vi "Elemente auswerten.vi"(7 "GObject (Eingang)":refnum<vi>, 8 "Fehler (Eingang, kein Fehler)":errorcluster, 9 "Sprachauswahl":u16, 10 "all rows":string[][](array[string]), 11 "ClassID":u32) -> (0 "error out":errorcluster, 1 "Sprachauswahl out":u16, 2 "all rows out":string[][](array[string]), 3 "ClassID out":u32, 4 "Cluster Elemente[]":refnum<vi>[](array[refnum]), 5 "Strings [4]":string[](array[string]))   [LabVIEW 2020, in "Sprachverwaltung.lvlib"]
uses:
  Sprachverwaltung.lvlib
panel:
  # "3 Generic \n4 Decoration \n5 Text \n6 Control \n7 ColorBox \n8 Boolean \n9 RefNum \n10 Variant \n11 Path \n12 ListBox \n13 Table \n14 Array \n15 Picture \n16 ActiveXContainer \n17 Numeric \n18 Digital \n19 NamedNumeric \n20 ColorRamp \n21 Slide \n22 GraphOrChart \n23 WaveformChart \n24 WaveformGraph \n25 IntensityChart \n26 IntensityGraph \n27 String \n28 IOName \n29 ComboBox \n30 Cluster \n31 Panel \n32 Knob \n33 NumWithScale \n34 Ring \n35 Enum \n36 GObject \n37 Plot \n38 Cursor \n39 NumericText \n40 Scale \n41 ColorScale \n42 GraphScale \n43 ColorGraphScale \n44 TypedRefNum \n45 OldKnobScale \n46 MCListbox \n47 MeasureData \n48 BVTag \n49 DAQName \n50 VISAName \n51 IVIName \n52 SlideScale \n54 Page \n55 TabControl \n56 ConPane"
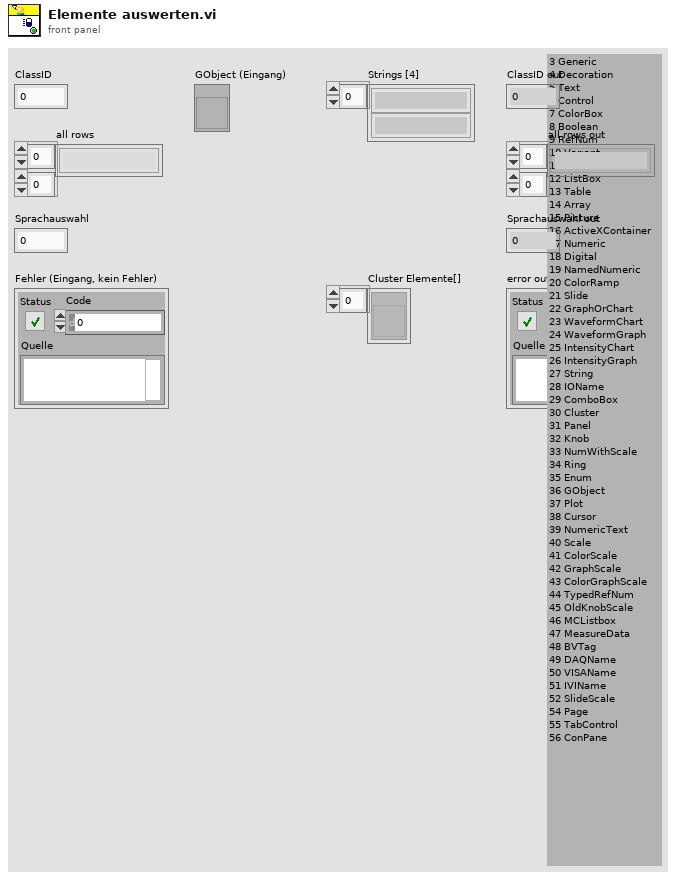
[diagram p1: front panel]
types:
  T1 = typedef "LVStringsAndValuesArrayTypeDef.ctl" = cluster{"String":string, "Value":ext}[]
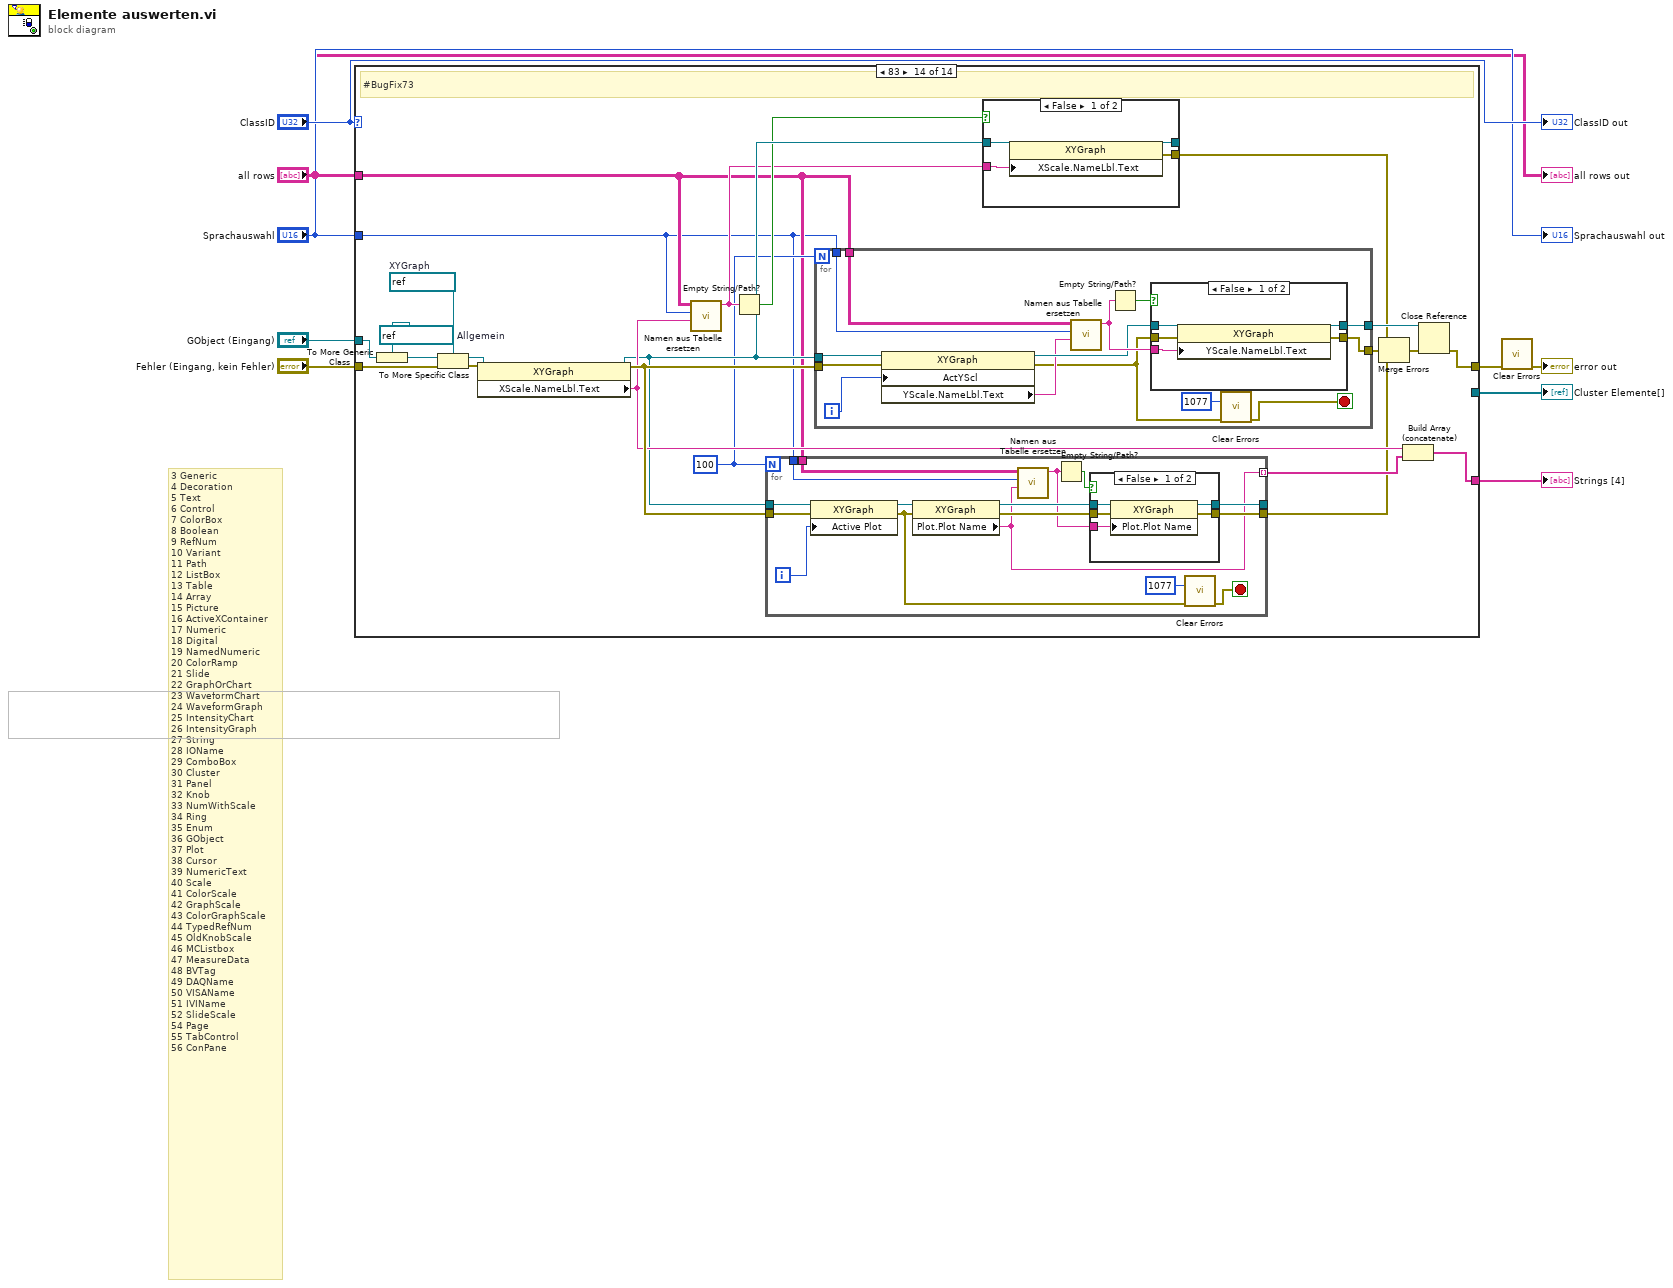
[diagram p0: block diagram]
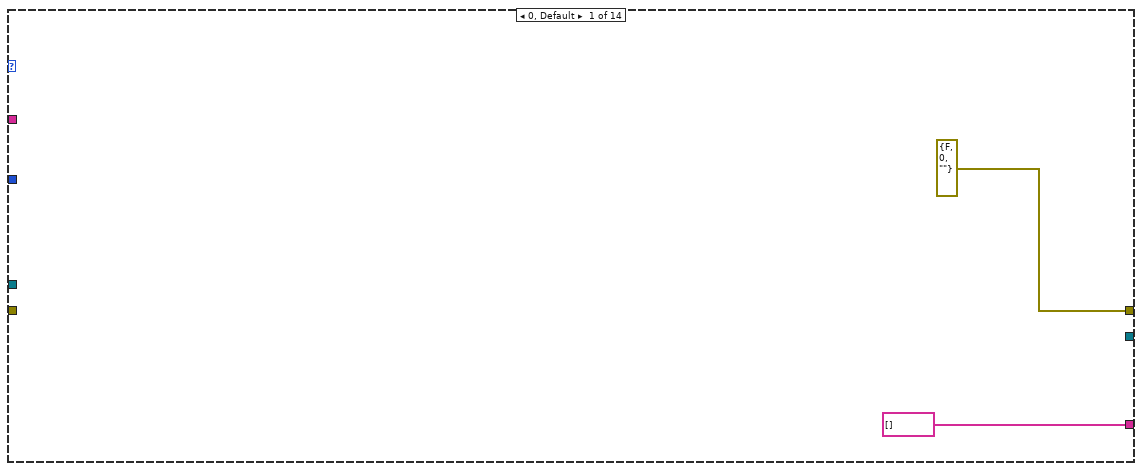
[diagram p2: hidden frame]
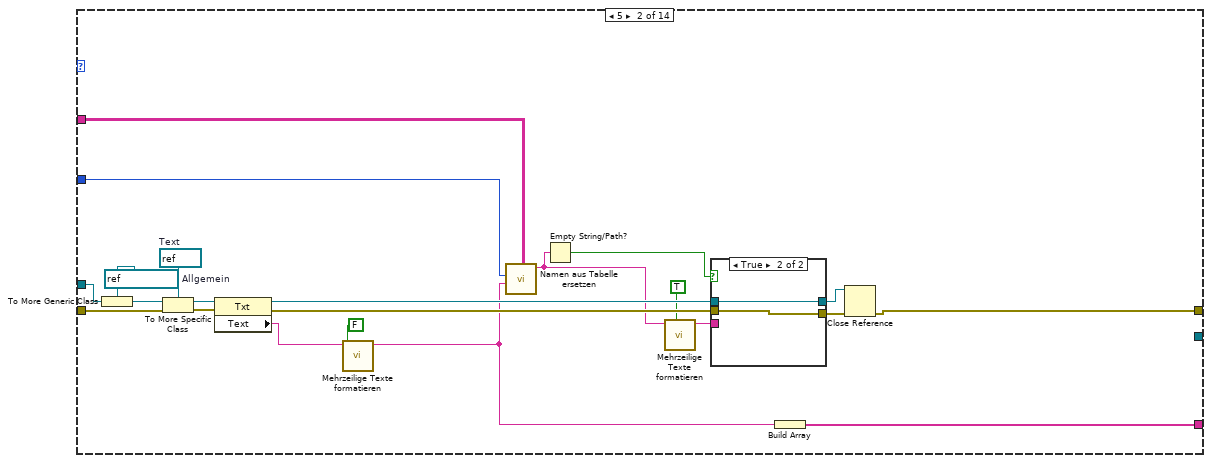
[diagram p3: hidden frame]
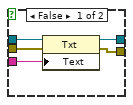
[diagram p4: hidden frame]
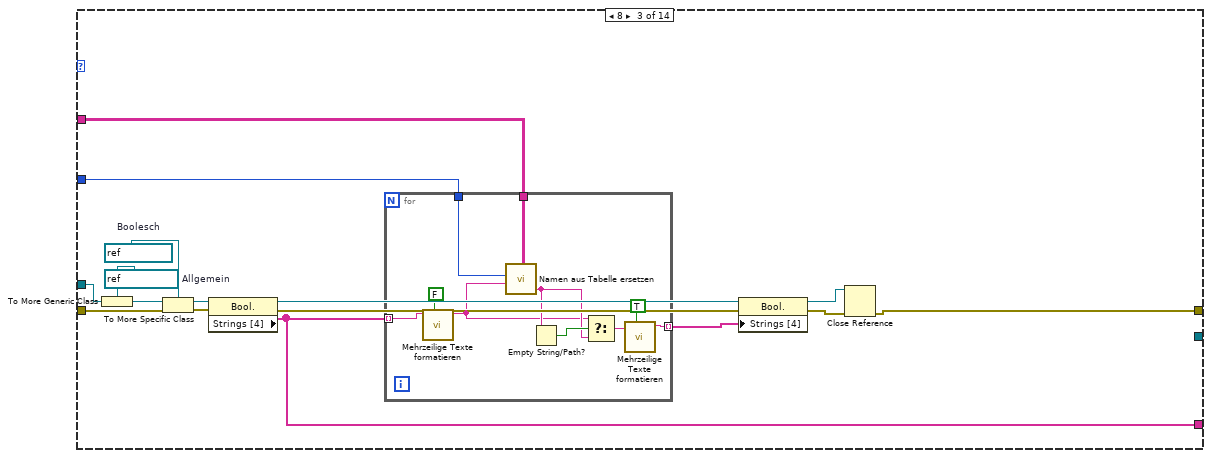
[diagram p5: hidden frame]
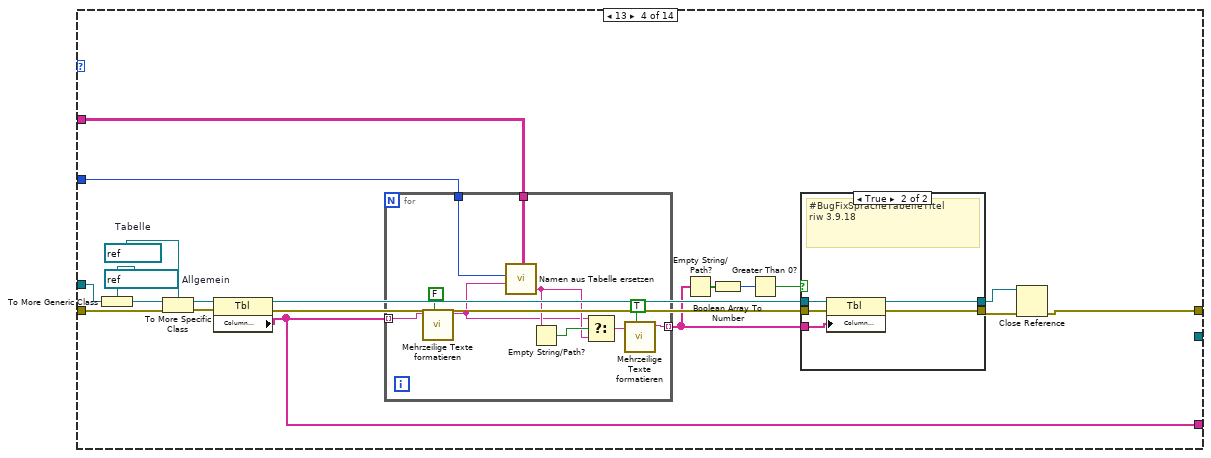
[diagram p6: hidden frame]
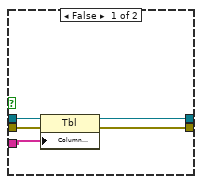
[diagram p7: hidden frame]
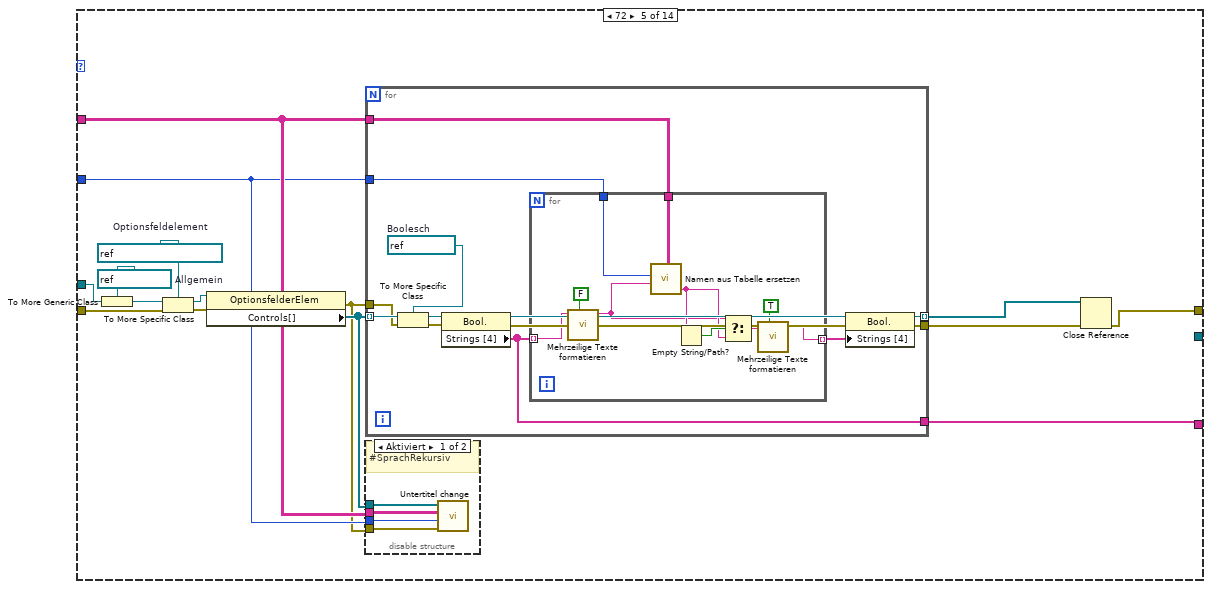
[diagram p8: hidden frame]
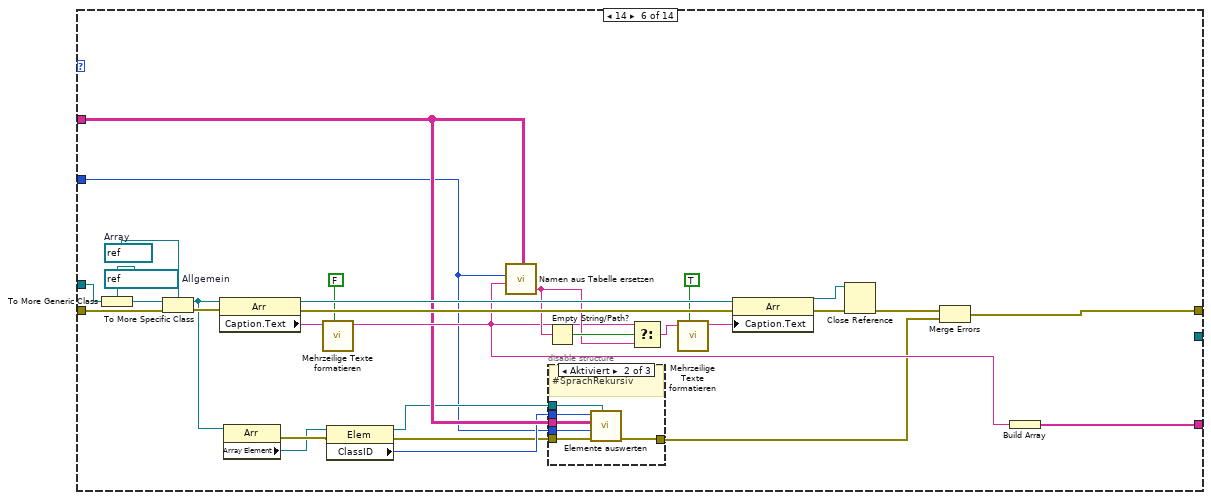
[diagram p10: hidden frame]
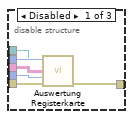
[diagram p11: hidden frame]
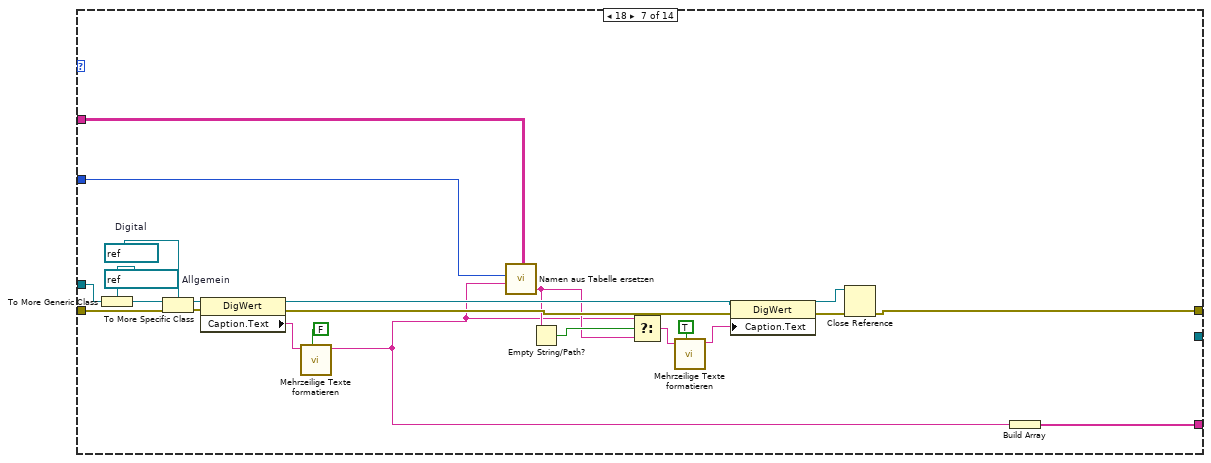
[diagram p13: hidden frame]
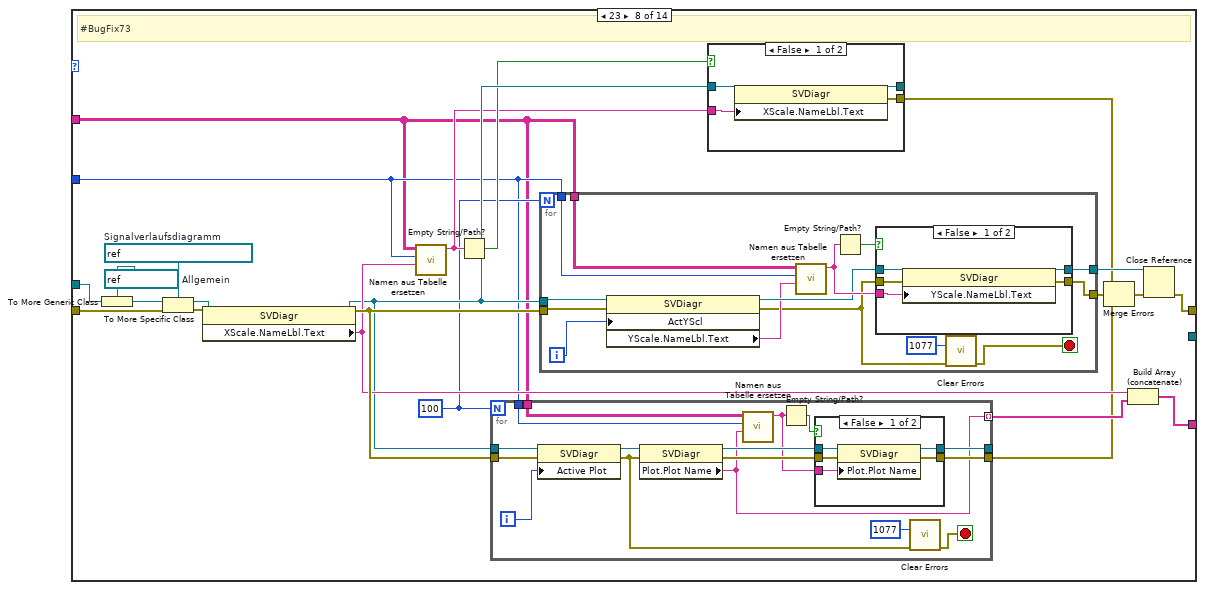
[diagram p14: hidden frame]
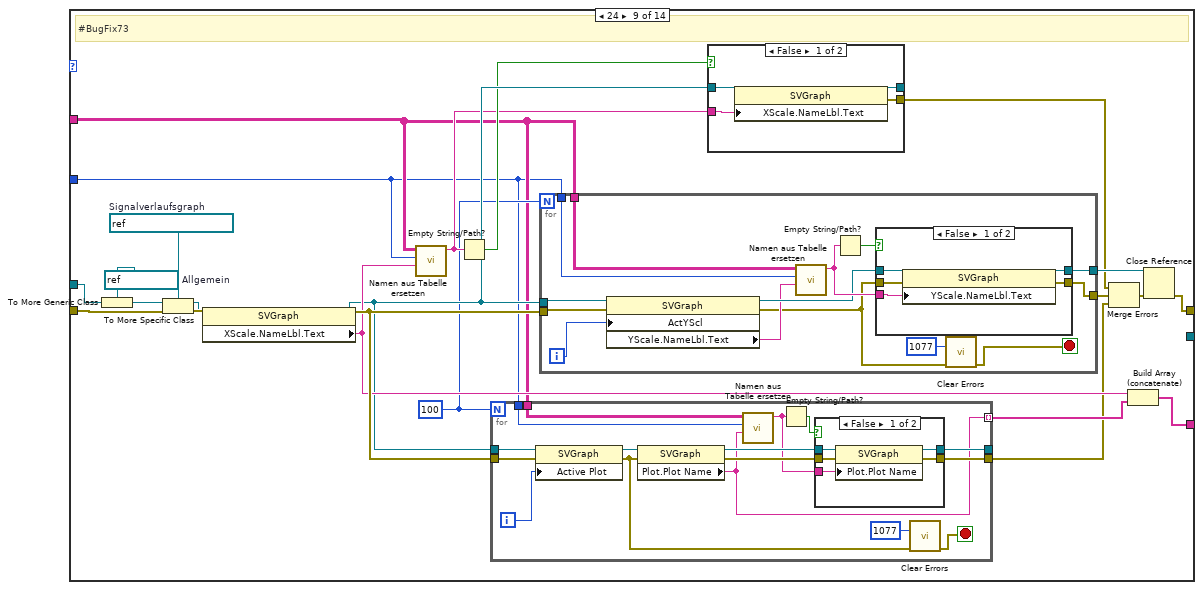
[diagram p18: hidden frame]
diagram:
  # "3 Generic \n4 Decoration \n5 Text \n6 Control \n7 ColorBox \n8 Boolean \n9 RefNum \n10 Variant \n11 Path \n12 ListBox \n13 Table \n14 Array \n15 Picture \n16 ActiveXContainer \n17 Numeric \n18 Digital \n19 NamedNumeric \n20 ColorRamp \n21 Slide \n22 GraphOrChart \n23 WaveformChart \n24 WaveformGraph \n25 IntensityChart \n26 IntensityGraph \n27 String \n28 IOName \n29 ComboBox \n30 Cluster \n31 Panel \n32 Knob \n33 NumWithScale \n34 Ring \n35 Enum \n36 GObject \n37 Plot \n38 Cursor \n39 NumericText \n40 Scale \n41 ColorScale \n42 GraphScale \n43 ColorGraphScale \n44 TypedRefNum \n45 OldKnobScale \n46 MCListbox \n47 MeasureData \n48 BVTag \n49 DAQName \n50 VISAName \n51 IVIName \n52 SlideScale \n54 Page \n55 TabControl \n56 ConPane"
  n1 = case shown="83" "ClassID" {
    tunnel: "GObject (Eingang)" -> [_ w33 w56 w85 w120 w177 w212 w218 w291 w373 w440 w482 w510 w530]
    tunnel: "Fehler (Eingang, kein Fehler)" -> [_ w30 w53 w82 w117 w174 w209 w219 w290 w370 w437 w479 w507 w535]
    tunnel: "all rows" -> [_ w26 w51 w80 w108 w156 w205 w220 w293 w361 w432 w471 w497 w534]
    tunnel: "Sprachauswahl" -> [_ w19 w50 w79 w107 w151 w204 w221 w292 w360 w431 w470 w498 w531]
    tunnel: [string[] [] ("Strings [4]") w18 w43 w73 w112 w166 w198 w216 w288 w366 w422 w458 w501 w533] -> w9
    tunnel: [_ _ _ _ _ _ _ _ _ w364 _ _ _ _] -> w3
    tunnel: [errorcluster {"status"=FALSE, "code"=0, "source"=""} ("error out") w21 w45 w74 w115 w149 w199 w217 w289 w358 w426 w466 w500 w532] -> w2
    frame 0, Default {
    }
    frame 5 {
      w29 = refnum<vi> refnum  # Text
      w32 = refnum<vi> refnum  # Allgemein
      n2 = To More Generic Class(target class=w32, reference=w33) -> (generic class reference=w31:refnum<vi>)
      n3 = To More Specific Class(target class=w29, reference=w31, error in=w30) -> (specific class reference=w28:refnum<vi>, error out=w27:errorcluster)
      n4 = property class="Txt"(reference=w28, error in=w27) -> (reference out=w24:refnum<vi>, error out=w25:errorcluster, "Text"=w17:string)
      n5 = call "Mehrzeilige Texte formatieren.vi"("Zurück formatieren"=FALSE, "string"=w17) -> ("result string"=w16:string)  [unwired: 9 in]
      n6 = call "Namen aus Tabelle ersetzen.vi"("Regulärer Ausdruck"=w16, "Sprachauswahl"=w19, "Tabelle"=w26) -> ("Übersetzung"=w13:string)  [unwired: 7 in, 1 out]
      n7 = Empty String/Path?(string/path=w13) -> (empty?=w20:bool)
      n8 = call "Mehrzeilige Texte formatieren.vi"("Zurück formatieren"=TRUE, "string"=w13) -> ("result string"=w12:string)  [unwired: 9 in]
      n9 = case shown="True" w20 {
        tunnel: w25 -> [w38 w39]
        tunnel: w24 -> [w37 w40]
        tunnel: w12 -> [w36 _]
        tunnel: [w35 w39] -> w23
        tunnel: [w34 w40] -> w22
        frame False {
          n10 = property class="Txt"(reference=w37, error in=w38, "Text"=w36) -> (reference out=w34:refnum<vi>, error out=w35:errorcluster)
        }
        frame True {
        }
      }
      n11 = Build Array(w16) -> (w18:string[])
      n12 = Close Reference(reference=w22, error in (no error)=w23) -> (error out=w21:errorcluster)
    }
    frame 8 {
      w52 = refnum<vi> refnum  # Boolesch
      w55 = refnum<vi> refnum  # Allgemein
      n13 = To More Generic Class(target class=w55, reference=w56) -> (generic class reference=w54:refnum<vi>)
      n14 = To More Specific Class(target class=w52, reference=w54, error in=w53) -> (specific class reference=w41:refnum<vi>, error out=w42:errorcluster)
      n15 = property class="Bool."(reference=w41, error in=w42) -> (reference out=w48:refnum<vi>, error out=w49:errorcluster, "Strings [4]"=w43:string[])
      n16 = for {
        tunnel: w43 -> [w61] mode=indexing
        tunnel: w51 -> [w66]
        tunnel: w50 -> [w65]
        tunnel: [w57] -> w44 mode=indexing
        n17 = call "Mehrzeilige Texte formatieren.vi"("Zurück formatieren"=FALSE, "string"=w61) -> ("result string"=w60:string)  [unwired: 9 in]
        n18 = call "Namen aus Tabelle ersetzen.vi"("Regulärer Ausdruck"=w60, "Sprachauswahl"=w65, "Tabelle"=w66) -> ("Übersetzung"=w63:string)  [unwired: 7 in, 1 out]
        n19 = Empty String/Path?(string/path=w63) -> (empty?=w64:bool)
        n20 = Select(t=w60, s=w64, f=w63) -> (s? t:f=w58:string)
        n21 = call "Mehrzeilige Texte formatieren.vi"("Zurück formatieren"=TRUE, "string"=w58) -> ("result string"=w57:string)  [unwired: 9 in]
      }
      n22 = property class="Bool."(reference=w48, error in=w49, "Strings [4]"=w44) -> (reference out=w46:refnum<vi>, error out=w47:errorcluster)
      n23 = Close Reference(reference=w46, error in (no error)=w47) -> (error out=w45:errorcluster)
    }
    frame 13 {
      w81 = refnum<vi> refnum  # Tabelle
      w84 = refnum<vi> refnum  # Allgemein
      n24 = To More Generic Class(target class=w84, reference=w85) -> (generic class reference=w83:refnum<vi>)
      n25 = To More Specific Class(target class=w81, reference=w83, error in=w82) -> (specific class reference=w71:refnum<vi>, error out=w72:errorcluster)
      n26 = property class="Tbl"(reference=w71, error in=w72) -> (reference out=w77:refnum<vi>, error out=w78:errorcluster, "Column Headers[]"=w73:string[])
      n27 = for {
        tunnel: w73 -> [w100] mode=indexing
        tunnel: w80 -> [w105]
        tunnel: w79 -> [w104]
        tunnel: [w96] -> w70 mode=indexing
        n28 = call "Mehrzeilige Texte formatieren.vi"("Zurück formatieren"=FALSE, "string"=w100) -> ("result string"=w99:string)  [unwired: 9 in]
        n29 = call "Namen aus Tabelle ersetzen.vi"("Regulärer Ausdruck"=w99, "Sprachauswahl"=w104, "Tabelle"=w105) -> ("Übersetzung"=w102:string)  [unwired: 7 in, 1 out]
        n30 = Empty String/Path?(string/path=w102) -> (empty?=w103:bool)
        n31 = Select(t=w99, s=w103, f=w102) -> (s? t:f=w97:string)
        n32 = call "Mehrzeilige Texte formatieren.vi"("Zurück formatieren"=TRUE, "string"=w97) -> ("result string"=w96:string)  [unwired: 9 in]
      }
      n33 = Empty String/Path?(string/path=w70) -> (empty?=w69:bool[])
      n34 = Boolean Array To Number(Boolean array=w69) -> (number=w68:u32)
      n35 = Greater Than 0?(x=w68) -> (x > 0?=w67:bool)
      n36 = case shown="True" w67 {
        tunnel: w78 -> [w90 w93]
        tunnel: w77 -> [w89 w95]
        tunnel: [w88 w92] -> w76
        tunnel: [w87 w94] -> w75
        tunnel: w70 -> [w86 w91]
        frame False {
          n37 = property class="Tbl"(reference=w89, error in=w90, "Column Headers[]"=w86) -> (reference out=w87:refnum<vi>, error out=w88:errorcluster)
        }
        frame True {
          # "#BugFixSpracheTabelleTitel\nriw 3.9.18"
          n38 = property class="Tbl"(reference=w95, error in=w93, "Column Headers[]"=w91) -> (reference out=w94:refnum<vi>, error out=w92:errorcluster)
        }
      }
      n39 = Close Reference(reference=w75, error in (no error)=w76) -> (error out=w74:errorcluster)
    }
    frame 72 {
      w116 = refnum<vi> refnum  # Optionsfeldelement
      w119 = refnum<vi> refnum  # Allgemein
      n40 = To More Generic Class(target class=w119, reference=w120) -> (generic class reference=w118:refnum<vi>)
      n41 = To More Specific Class(target class=w116, reference=w118, error in=w117) -> (specific class reference=w113:refnum<vi>, error out=w114:errorcluster)
      n42 = property class="OptionsfelderElem"(reference=w113, error in=w114) -> (error out=w106:errorcluster, "Controls[]"=w109:refnum<vi>[])  [unwired: 1 out]
      n43 = for {
        tunnel: w108 -> [w127]
        tunnel: w107 -> [w126]
        tunnel: w109 -> [w128] mode=indexing
        tunnel: [w135] -> w112
        tunnel: w106 -> [w125]
        tunnel: [w130] -> w111
        tunnel: [w129] -> w110 mode=indexing
        w137 = refnum<vi> refnum  # Boolesch
        n44 = To More Specific Class(target class=w137, reference=w128, error in=w125) -> (specific class reference=w136:refnum<vi>, error out=w134:errorcluster)
        n45 = property class="Bool."(reference=w136, error in=w134) -> (reference out=w133:refnum<vi>, error out=w132:errorcluster, "Strings [4]"=w135:string[])
        n46 = for {
          tunnel: w127 -> [w147]
          tunnel: w126 -> [w146]
          tunnel: [w139] -> w131 mode=indexing
          tunnel: w135 -> [w138] mode=indexing
          n47 = call "Mehrzeilige Texte formatieren.vi"("Zurück formatieren"=FALSE, "string"=w138) -> ("result string"=w142:string)  [unwired: 9 in]
          n48 = call "Namen aus Tabelle ersetzen.vi"("Regulärer Ausdruck"=w142, "Sprachauswahl"=w146, "Tabelle"=w147) -> ("Übersetzung"=w144:string)  [unwired: 7 in, 1 out]
          n49 = Empty String/Path?(string/path=w144) -> (empty?=w145:bool)
          n50 = Select(t=w142, s=w145, f=w144) -> (s? t:f=w140:string)
          n51 = call "Mehrzeilige Texte formatieren.vi"("Zurück formatieren"=TRUE, "string"=w140) -> ("result string"=w139:string)  [unwired: 9 in]
        }
        n52 = property class="Bool."(reference=w133, error in=w132, "Strings [4]"=w131) -> (reference out=w129:refnum<vi>, error out=w130:errorcluster)
      }
      n53 = disable-structure shown="Aktiviert" {
        disable-tunnel: w109 -> [w124 _]
        disable-tunnel: w108 -> [w123 _]
        disable-tunnel: w107 -> [w122 _]
        disable-tunnel: w106 -> [w121 _]
        frame Enabled {
          # "#SprachRekursiv"
          n54 = call "Untertitel change.vi"("Fehler (Eingang, kein Fehler)"=w121, "Sprachauswahl"=w122, "Sprachdatei"=w123, "Controls[]"=w124) -> ()  [unwired: 5 in, 3 out]
        }
        frame Disabled {
        }
      }
      n55 = Close Reference(reference=w110, error in (no error)=w111) -> (error out=w115:errorcluster)
    }
    frame 14 {
      w173 = refnum<vi> refnum  # Array
      w176 = refnum<vi> refnum  # Allgemein
      n56 = To More Generic Class(target class=w176, reference=w177) -> (generic class reference=w175:refnum<vi>)
      n57 = To More Specific Class(target class=w173, reference=w175, error in=w174) -> (specific class reference=w157:refnum<vi>, error out=w172:errorcluster)
      n58 = property class="Arr"(reference=w157, error in=w172) -> (reference out=w170:refnum<vi>, error out=w171:errorcluster, "Caption.Text"=w162:string)
      n59 = property class="Arr"(reference=w157) -> (error out=w155:errorcluster, "Array Element"=w154:refnum<vi>)  [unwired: 1 in, 1 out]
      n60 = call "Mehrzeilige Texte formatieren.vi"("Zurück formatieren"=FALSE, "string"=w162) -> ("result string"=w161:string)  [unwired: 9 in]
      n61 = property class="Elem"(reference=w154, error in=w155) -> (reference out=w152:refnum<vi>, error out=w150:errorcluster, "ClassID"=w153:u32)
      n62 = call "Namen aus Tabelle ersetzen.vi"("Regulärer Ausdruck"=w161, "Sprachauswahl"=w151, "Tabelle"=w156) -> ("Übersetzung"=w164:string)  [unwired: 7 in, 1 out]
      n63 = Empty String/Path?(string/path=w164) -> (empty?=w165:bool)
      n64 = disable-structure shown="Aktiviert" {
        disable-tunnel: w156 -> [w183 w189 _]
        disable-tunnel: w153 -> [w182 w185 _]
        disable-tunnel: w152 -> [w181 w184 _]
        disable-tunnel: w151 -> [w180 w188 _]
        disable-tunnel: w150 -> [w179 w187 _]
        disable-tunnel: [w178 w186 _] -> w148
        frame Disabled {
          n65 = call "Auswertung Registerkarte.vi"("GObject (Eingang)"=w181, "ClassID"=w182, "all rows"=w183, "Sprachauswahl"=w180, "Fehler (Eingang, kein Fehler)"=w179) -> ("error out"=w178:errorcluster)  [unwired: 9 in, 1 out]
        }
        frame Enabled {
          # "#SprachRekursiv"
          n66 = call "Elemente auswerten.vi"("GObject (Eingang)"=w184, "Fehler (Eingang, kein Fehler)"=w187, "Sprachauswahl"=w188, "all rows"=w189, "ClassID"=w185) -> ("error out"=w186:errorcluster)  [unwired: 1 in, 5 out]
        }
        frame Disabled {
        }
      }
      n67 = Select(t=w161, s=w165, f=w164) -> (s? t:f=w159:string)
      n68 = call "Mehrzeilige Texte formatieren.vi"("Zurück formatieren"=TRUE, "string"=w159) -> ("result string"=w158:string)  [unwired: 9 in]
      n69 = property class="Arr"(reference=w170, error in=w171, "Caption.Text"=w158) -> (reference out=w168:refnum<vi>, error out=w169:errorcluster)
      n70 = Close Reference(reference=w168, error in (no error)=w169) -> (error out=w167:errorcluster)
      n71 = Merge Errors(w167, w148) -> (w149:errorcluster)
      n72 = Build Array(w161) -> (w166:string[])
    }
    frame 18 {
      w208 = refnum<vi> refnum  # Digital
      w211 = refnum<vi> refnum  # Allgemein
      n73 = To More Generic Class(target class=w211, reference=w212) -> (generic class reference=w210:refnum<vi>)
      n74 = To More Specific Class(target class=w208, reference=w210, error in=w209) -> (specific class reference=w207:refnum<vi>, error out=w206:errorcluster)
      n75 = property class="DigWert"(reference=w207, error in=w206) -> (reference out=w202:refnum<vi>, error out=w203:errorcluster, "Caption.Text"=w194:string)
      n76 = call "Mehrzeilige Texte formatieren.vi"("Zurück formatieren"=FALSE, "string"=w194) -> ("result string"=w193:string)  [unwired: 9 in]
      n77 = call "Namen aus Tabelle ersetzen.vi"("Regulärer Ausdruck"=w193, "Sprachauswahl"=w204, "Tabelle"=w205) -> ("Übersetzung"=w196:string)  [unwired: 7 in, 1 out]
      n78 = Empty String/Path?(string/path=w196) -> (empty?=w197:bool)
      n79 = Select(t=w193, s=w197, f=w196) -> (s? t:f=w191:string)
      n80 = call "Mehrzeilige Texte formatieren.vi"("Zurück formatieren"=TRUE, "string"=w191) -> ("result string"=w190:string)  [unwired: 9 in]
      n81 = property class="DigWert"(reference=w202, error in=w203, "Caption.Text"=w190) -> (reference out=w200:refnum<vi>, error out=w201:errorcluster)
      n82 = Close Reference(reference=w200, error in (no error)=w201) -> (error out=w199:errorcluster)
      n83 = Build Array(w193) -> (w198:string[])
    }
    frame 23 {
      w222 = 100
      w233 = refnum<vi> refnum  # Signalverlaufsdiagramm
      w235 = refnum<vi> refnum  # Allgemein
      # "#BugFix73"
      n84 = To More Generic Class(target class=w235, reference=w218) -> (generic class reference=w234:refnum<vi>)
      n85 = To More Specific Class(target class=w233, reference=w234, error in=w219) -> (specific class reference=w232:refnum<vi>, error out=w231:errorcluster)
      n86 = property class="SVDiagr"(reference=w232, error in=w231) -> (reference out=w225:refnum<vi>, error out=w230:errorcluster, "XScale.NameLbl.Text"=w226:string)
      n87 = call "Namen aus Tabelle ersetzen.vi"("Regulärer Ausdruck"=w226, "Sprachauswahl"=w221, "Tabelle"=w220) -> ("Übersetzung"=w223:string)  [unwired: 7 in, 1 out]
      n88 = Empty String/Path?(string/path=w223) -> (empty?=w224:bool)
      n89 = for {
        N: w222 -> [_]
        tunnel: w225 -> [w256]
        tunnel: w230 -> [w253]
        tunnel: w220 -> [w252]
        tunnel: w221 -> [w251]
        tunnel: [w247] -> _
        tunnel: [w246] -> w214
        tunnel: [w244] -> w227 mode=indexing
        i -> [w255]
        stop <- w242 stop-if-true
        n90 = property class="SVDiagr"(reference=w256, error in=w253, "Active Plot"=w255) -> (reference out=w254:refnum<vi>, error out=w241:errorcluster)
        n91 = property class="SVDiagr"(reference=w254, error in=w241) -> (reference out=w250:refnum<vi>, error out=w249:errorcluster, "Plot.Plot Name"=w244:string)
        n92 = call "Namen aus Tabelle ersetzen.vi"("Regulärer Ausdruck"=w244, "Sprachauswahl"=w251, "Tabelle"=w252) -> ("Übersetzung"=w245:string)  [unwired: 7 in, 1 out]
        n93 = Empty String/Path?(string/path=w245) -> (empty?=w248:bool)
        n94 = case shown="False" w248 {
          tunnel: w250 -> [w261 w263]
          tunnel: w249 -> [w260 w262]
          tunnel: [w259 w263] -> w247
          tunnel: [w258 w262] -> w246
          tunnel: w245 -> [w257 _]
          frame False {
            n95 = property class="SVDiagr"(reference=w261, error in=w260, "Plot.Plot Name"=w257) -> (reference out=w259:refnum<vi>, error out=w258:errorcluster)
          }
          frame True {
          }
        }
        n96 = call <vilib>:"Clear Errors.vi"("error in (no error)"=w241, "specific error code to clear (0: all)"=1077) -> ("error out"=w242:errorcluster)  [unwired: 4 in, 1 out]
      }
      n97 = for {
        N: w222 -> [_]
        tunnel: w220 -> [w277]
        tunnel: w221 -> [w272]
        tunnel: w225 -> [w270]
        tunnel: w230 -> [w271]
        tunnel: [w274] -> w229
        tunnel: [w273] -> w228
        i -> [w268]
        stop <- w266 stop-if-true
        n98 = property class="SVDiagr"(reference=w270, error in=w271, "ActYScl"=w268) -> (reference out=w269:refnum<vi>, error out=w265:errorcluster, "YScale.NameLbl.Text"=w267:string)
        n99 = call "Namen aus Tabelle ersetzen.vi"("Regulärer Ausdruck"=w267, "Sprachauswahl"=w272, "Tabelle"=w277) -> ("Übersetzung"=w275:string)  [unwired: 7 in, 1 out]
        n100 = Empty String/Path?(string/path=w275) -> (empty?=w276:bool)
        n101 = case shown="False" w276 {
          tunnel: w265 -> [w282 w283]
          tunnel: w269 -> [w281 w284]
          tunnel: [w280 w283] -> w273
          tunnel: [w279 w284] -> w274
          tunnel: w275 -> [w278 _]
          frame False {
            n102 = property class="SVDiagr"(reference=w281, error in=w282, "YScale.NameLbl.Text"=w278) -> (reference out=w279:refnum<vi>, error out=w280:errorcluster)
          }
          frame True {
          }
        }
        n103 = call <vilib>:"Clear Errors.vi"("error in (no error)"=w265, "specific error code to clear (0: all)"=1077) -> ("error out"=w266:errorcluster)  [unwired: 4 in, 1 out]
      }
      n104 = case shown="False" w224 {
        tunnel: w225 -> [w239 w240]
        tunnel: [w238 _] -> w213
        tunnel: [w237 w240] -> _
        tunnel: w223 -> [w236 _]
        frame False {
          n105 = property class="SVDiagr"(reference=w239, "XScale.NameLbl.Text"=w236) -> (reference out=w237:refnum<vi>, error out=w238:errorcluster)  [unwired: 1 in]
        }
        frame True {
        }
      }
      n106 = Merge Errors(w213, w228, w214) -> (w215:errorcluster)
      n107 = Build Array (concatenate)(w226, w227) -> (w216:string[])
      n108 = Close Reference(reference=w229, error in (no error)=w215) -> (error out=w217:errorcluster)
    }
    frame 24 {
      w295 = refnum<vi> refnum  # Signalverlaufsgraph
      w296 = 100
      w307 = refnum<vi> refnum  # Allgemein
      # "#BugFix73"
      n109 = To More Generic Class(target class=w307, reference=w291) -> (generic class reference=w306:refnum<vi>)
      n110 = To More Specific Class(target class=w295, reference=w306, error in=w290) -> (specific class reference=w294:refnum<vi>, error out=w305:errorcluster)
      n111 = property class="SVGraph"(reference=w294, error in=w305) -> (reference out=w299:refnum<vi>, error out=w304:errorcluster, "XScale.NameLbl.Text"=w300:string)
      n112 = call "Namen aus Tabelle ersetzen.vi"("Regulärer Ausdruck"=w300, "Sprachauswahl"=w292, "Tabelle"=w293) -> ("Übersetzung"=w297:string)  [unwired: 7 in, 1 out]
      n113 = Empty String/Path?(string/path=w297) -> (empty?=w298:bool)
      n114 = for {
        N: w296 -> [_]
        tunnel: w299 -> [w328]
        tunnel: w304 -> [w325]
        tunnel: w293 -> [w324]
        tunnel: w292 -> [w323]
        tunnel: [w319] -> _
        tunnel: [w318] -> w286
        tunnel: [w316] -> w301 mode=indexing
        i -> [w327]
        stop <- w314 stop-if-true
        n115 = property class="SVGraph"(reference=w328, error in=w325, "Active Plot"=w327) -> (reference out=w326:refnum<vi>, error out=w313:errorcluster)
        n116 = property class="SVGraph"(reference=w326, error in=w313) -> (reference out=w322:refnum<vi>, error out=w321:errorcluster, "Plot.Plot Name"=w316:string)
        n117 = call "Namen aus Tabelle ersetzen.vi"("Regulärer Ausdruck"=w316, "Sprachauswahl"=w323, "Tabelle"=w324) -> ("Übersetzung"=w317:string)  [unwired: 7 in, 1 out]
        n118 = Empty String/Path?(string/path=w317) -> (empty?=w320:bool)
        n119 = case shown="False" w320 {
          tunnel: w322 -> [w333 w335]
          tunnel: w321 -> [w332 w334]
          tunnel: [w331 w335] -> w319
          tunnel: [w330 w334] -> w318
          tunnel: w317 -> [w329 _]
          frame False {
            n120 = property class="SVGraph"(reference=w333, error in=w332, "Plot.Plot Name"=w329) -> (reference out=w331:refnum<vi>, error out=w330:errorcluster)
          }
          frame True {
          }
        }
        n121 = call <vilib>:"Clear Errors.vi"("error in (no error)"=w313, "specific error code to clear (0: all)"=1077) -> ("error out"=w314:errorcluster)  [unwired: 4 in, 1 out]
      }
      n122 = for {
        N: w296 -> [_]
        tunnel: w293 -> [w349]
        tunnel: w292 -> [w344]
        tunnel: w299 -> [w342]
        tunnel: w304 -> [w343]
        tunnel: [w346] -> w303
        tunnel: [w345] -> w302
        i -> [w340]
        stop <- w338 stop-if-true
        n123 = property class="SVGraph"(reference=w342, error in=w343, "ActYScl"=w340) -> (reference out=w341:refnum<vi>, error out=w337:errorcluster, "YScale.NameLbl.Text"=w339:string)
        n124 = call "Namen aus Tabelle ersetzen.vi"("Regulärer Ausdruck"=w339, "Sprachauswahl"=w344, "Tabelle"=w349) -> ("Übersetzung"=w347:string)  [unwired: 7 in, 1 out]
        n125 = Empty String/Path?(string/path=w347) -> (empty?=w348:bool)
        n126 = case shown="False" w348 {
          tunnel: w337 -> [w354 w355]
          tunnel: w341 -> [w353 w356]
          tunnel: [w352 w355] -> w345
          tunnel: [w351 w356] -> w346
          tunnel: w347 -> [w350 _]
          frame False {
            n127 = property class="SVGraph"(reference=w353, error in=w354, "YScale.NameLbl.Text"=w350) -> (reference out=w351:refnum<vi>, error out=w352:errorcluster)
          }
          frame True {
          }
        }
        n128 = call <vilib>:"Clear Errors.vi"("error in (no error)"=w337, "specific error code to clear (0: all)"=1077) -> ("error out"=w338:errorcluster)  [unwired: 4 in, 1 out]
      }
      n129 = case shown="False" w298 {
        tunnel: w299 -> [w311 w312]
        tunnel: [w310 _] -> w285
        tunnel: [w309 w312] -> _
        tunnel: w297 -> [w308 _]
        frame False {
          n130 = property class="SVGraph"(reference=w311, "XScale.NameLbl.Text"=w308) -> (reference out=w309:refnum<vi>, error out=w310:errorcluster)  [unwired: 1 in]
        }
        frame True {
        }
      }
      n131 = Merge Errors(w285, w302, w286) -> (w287:errorcluster)
      n132 = Build Array (concatenate)(w300, w301) -> (w288:string[])
      n133 = Close Reference(reference=w303, error in (no error)=w287) -> (error out=w289:errorcluster)
    }
    frame 30 {
      w369 = refnum<vi> refnum  # Cluster
      w372 = refnum<vi> refnum  # Allgemein
      n134 = To More Generic Class(target class=w372, reference=w373) -> (generic class reference=w371:refnum<vi>)
      n135 = To More Specific Class(target class=w369, reference=w371, error in=w370) -> (specific class reference=w368:refnum<vi>, error out=w367:errorcluster)
      n136 = property class="Cluster"(reference=w368, error in=w367) -> (reference out=w365:refnum<vi>, error out=w359:errorcluster, "Controls[]"=w364:refnum<vi>[], "AllObjs[]"=w362:refnum<vi>[])
      n137 = for {
        tunnel: w361 -> [w399]
        tunnel: w359 -> [w403]
        tunnel: w365 -> [_]
        tunnel: w360 -> [w401]
        tunnel: w364 -> [w400] mode=indexing
        tunnel: [w406] -> w366 mode=indexing
        tunnel: [w410] -> w363
        n138 = property class="Elem"(reference=w400, error in=w403) -> (reference out=w411:refnum<vi>, error out=w402:errorcluster, "Caption.Text"=w407:string)
        n139 = call "Mehrzeilige Texte formatieren.vi"("Zurück formatieren"=FALSE, "string"=w407) -> ("result string"=w406:string)  [unwired: 9 in]
        n140 = call "Namen aus Tabelle ersetzen.vi"("Regulärer Ausdruck"=w406, "Sprachauswahl"=w401, "Tabelle"=w399) -> ("Übersetzung"=w405:string)  [unwired: 7 in, 1 out]
        n141 = Empty String/Path?(string/path=w405) -> (empty?=w412:bool)
        n142 = call "Mehrzeilige Texte formatieren.vi"("Zurück formatieren"=TRUE, "string"=w405) -> ("result string"=w404:string)  [unwired: 9 in]
        n143 = case shown="False" w412 {
          tunnel: w402 -> [w419 w420]
          tunnel: w411 -> [w418 w421]
          tunnel: w404 -> [w417 _]
          tunnel: [w416 w420] -> w414
          tunnel: [w415 w421] -> w413
          frame False {
            n144 = property class="Elem"(reference=w418, error in=w419, "Caption.Text"=w417) -> (reference out=w415:refnum<vi>, error out=w416:errorcluster)
          }
          frame True {
          }
        }
        n145 = Close Reference(reference=w413, error in (no error)=w414) -> (error out=w410:errorcluster)
      }
      n146 = for {
        tunnel: w362 -> [w385] mode=indexing
        tunnel: w361 -> [w382]
        tunnel: w360 -> [w384]
        shift-right: [w381] -> w357
        shift-left: w359 -> [w380]
        # "#LudicrousMode"
        n147 = property class="GObj"(reference=w385, error in=w380) -> (reference out=w378:refnum<vi>, error out=w379:errorcluster, "ClassID"=w377:u32)
        n148 = call "Elemente auswerten.vi"("GObject (Eingang)"=w378, "Fehler (Eingang, kein Fehler)"=w379, "Sprachauswahl"=w384, "all rows"=w382, "ClassID"=w377) -> ("error out"=w383:errorcluster, "Sprachauswahl out"=w376:u16, "all rows out"=w374:string[][], "Cluster Elemente[]"=w375:refnum<vi>[])  [unwired: 1 in, 2 out]
        n149 = disable-structure shown="Deaktiviert" {
          disable-tunnel: w375 -> [w390 _]
          disable-tunnel: w376 -> [w389 _]
          disable-tunnel: w383 -> [w388 w398]
          disable-tunnel: w374 -> [w387 _]
          disable-tunnel: [w386 w398] -> w381
          frame Disabled {
            n150 = for {
              tunnel: w387 -> [w397]
              tunnel: w389 -> [w394]
              tunnel: w390 -> [w395] mode=indexing
              shift-right: [w392] -> w386
              shift-left: w388 -> [w396]
              n151 = property class="Elem"(reference=w395) -> (reference out=w391:refnum<vi>, "ClassID"=w393:u32)  [unwired: 1 in, 1 out]
              n152 = call "Elemente auswerten.vi"("GObject (Eingang)"=w391, "Fehler (Eingang, kein Fehler)"=w396, "Sprachauswahl"=w394, "all rows"=w397, "ClassID"=w393) -> ("error out"=w392:errorcluster)  [unwired: 1 in, 5 out]
            }
          }
          frame Enabled {
          }
        }
      }
      n153 = Merge Errors(w363, w357) -> (w358:errorcluster)
    }
    frame 34 {
      w436 = refnum<vi> refnum  # Ring
      w439 = refnum<vi> refnum  # Allgemein
      n154 = To More Generic Class(target class=w439, reference=w440) -> (generic class reference=w438:refnum<vi>)
      n155 = To More Specific Class(target class=w436, reference=w438, error in=w437) -> (specific class reference=w435:refnum<vi>, error out=w434:errorcluster)
      n156 = property class="Ring"(reference=w435, error in=w434) -> (reference out=w429:refnum<vi>, error out=w430:errorcluster, "StringsAndValues[]"=w433:T1)
      n157 = for {
        tunnel: w433 -> [w452] mode=indexing
        tunnel: w432 -> [w457]
        tunnel: w431 -> [w449]
        tunnel: [w450] -> w425 mode=indexing
        shift-right: [w455] -> w423
        shift-left: FALSE -> [w454]
        tunnel: [w448] -> w422 mode=indexing
        n158 = Unbundle By Name(w452) -> ("String"=w448:string)
        n159 = call "Namen aus Tabelle ersetzen.vi"("Regulärer Ausdruck"=w448, "Sprachauswahl"=w449, "Tabelle"=w457) -> ("Übersetzung"=w451:string)  [unwired: 7 in, 1 out]
        n160 = Empty String/Path?(string/path=w451) -> (empty?=w456:bool)
        n161 = Bundle By Name(cluster=w452, "String"=w451) -> (w450:cluster{"String":string, "Value":ext})
        n162 = Select(t=TRUE, s=w456, f=w454) -> (s? t:f=w455:bool)
      }
      n163 = case shown="False" w423 {
        tunnel: w430 -> [w445 w446]
        tunnel: w429 -> [w444 w447]
        tunnel: w425 -> [w443 _]
        tunnel: [w442 w446] -> w428
        tunnel: [w441 w447] -> w427
        frame False {
          n164 = property class="Ring"(reference=w444, error in=w445, "StringsAndValues[]"=w443) -> (reference out=w441:refnum<vi>, error out=w442:errorcluster)
        }
        frame True {
        }
      }
      n165 = Close Reference(reference=w427, error in (no error)=w428) -> (error out=w426:errorcluster)
    }
    frame 46 {
      w478 = refnum<vi> refnum  # MehrspaltigesListenfeld
      w481 = refnum<vi> refnum  # Allgemein
      # "Eventuell die komplette Casestruktur mit allen funktionen einbauen?!!"
      n166 = To More Generic Class(target class=w481, reference=w482) -> (generic class reference=w480:refnum<vi>)
      n167 = To More Specific Class(target class=w478, reference=w480, error in=w479) -> (specific class reference=w472:refnum<vi>, error out=w477:errorcluster)
      n168 = property class="MehrSpaltFeld"(reference=w472, error in=w477) -> (reference out=w474:refnum<vi>, error out=w473:errorcluster, "RowHdrs[]"=w460:string[])
      n169 = property class="MehrSpaltFeld"(reference=w472) -> (reference out=w469:refnum<vi>, error out=w468:errorcluster, "ColHdrString"=w459:string[])  [unwired: 1 in]
      n170 = Build Array (concatenate)(w460, w459) -> (w458:string[])
      n171 = for {
        tunnel: w471 -> [w494]
        tunnel: w470 -> [w493]
        tunnel: w460 -> [w491] mode=indexing
        tunnel: [w489] -> w475 mode=indexing
        n172 = call "Namen aus Tabelle ersetzen.vi"("Regulärer Ausdruck"=w491, "Sprachauswahl"=w493, "Tabelle"=w494) -> ("Übersetzung"=w490:string)  [unwired: 7 in, 1 out]
        n173 = Empty String/Path?(string/path=w490) -> (empty?=w492:bool)
        n174 = Select(t=w491, s=w492, f=w490) -> (s? t:f=w489:string)
      }
      n175 = for {
        tunnel: w471 -> [w488]
        tunnel: w470 -> [w487]
        tunnel: w459 -> [w483] mode=indexing
        tunnel: [w484] -> w467 mode=indexing
        n176 = call "Namen aus Tabelle ersetzen.vi"("Regulärer Ausdruck"=w483, "Sprachauswahl"=w487, "Tabelle"=w488) -> ("Übersetzung"=w485:string)  [unwired: 7 in, 1 out]
        n177 = Empty String/Path?(string/path=w485) -> (empty?=w486:bool)
        n178 = Select(t=w483, s=w486, f=w485) -> (s? t:f=w484:string)
      }
      n179 = property class="MehrSpaltFeld"(reference=w469, error in=w468, "ColHdrString"=w467) -> (reference out=w462:refnum<vi>, error out=w464:errorcluster)
      n180 = property class="MehrSpaltFeld"(reference=w474, error in=w473, "RowHdrs[]"=w475) -> (reference out=w461:refnum<vi>, error out=w465:errorcluster)
      n181 = Merge Errors(w465, w464) -> (w463:errorcluster)
      n182 = Close Reference(reference=w461, error in (no error)=w463) -> (error out=w466:errorcluster)
      n183 = Close Reference(reference=w462, error in (no error)=w463) -> (error out=w476:errorcluster)
      n184 = call <vilib>:"Clear Errors.vi"("error in (no error)"=w476) -> ()  [unwired: 5 in, 2 out]
    }
    frame 55 {
      w506 = refnum<vi> refnum  # Registerkartenelement
      w509 = refnum<vi> refnum  # Allgemein
      # "mit RKUntertitel schon - riw 11.07.2018 #BugFixSpracheRegisterkarten"
      # "Funktioniert nicht!!"
      n185 = To More Generic Class(target class=w509, reference=w510) -> (generic class reference=w508:refnum<vi>)
      n186 = To More Specific Class(target class=w506, reference=w508, error in=w507) -> (specific class reference=w505:refnum<vi>, error out=w504:errorcluster)
      n187 = property class="RKElem"(reference=w505, error in=w504) -> (error out=w496:errorcluster, "Pages"=w499:refnum<vi>[])  [unwired: 1 out]
      n188 = call "Registerkartenverwaltung.vi"("Fehler (Eingang, kein Fehler)"=w496, "Sprachauswahl"=w498, "all rows"=w497, "Seiten"=w499) -> ("error out"=w495:errorcluster)  [unwired: 7 in]
      n189 = for {
        tunnel: w495 -> [w521]
        tunnel: w499 -> [w520] mode=indexing
        tunnel: w498 -> [w514]
        tunnel: w497 -> [w519]
        tunnel: [w516] -> w503
        tunnel: [w515] -> w502
        tunnel: [w513] -> w501 mode=indexing
        n190 = property class="Seite"(reference=w520, error in=w521) -> (reference out=w512:refnum<vi>, error out=w518:errorcluster, "TabCaption"=w513:string)
        n191 = call "Namen aus Tabelle ersetzen.vi"("Regulärer Ausdruck"=w513, "Sprachauswahl"=w514, "Tabelle"=w519) -> ("Übersetzung"=w517:string)  [unwired: 7 in, 1 out]
        n192 = Empty String/Path?(string/path=w517) -> (empty?=w511:bool)
        n193 = case shown="False" w511 {
          tunnel: w518 -> [w524 w528]
          tunnel: w512 -> [w527 w529]
          tunnel: [w525 w528] -> w515
          tunnel: [w526 w529] -> w516
          tunnel: w517 -> [w523 _]
          frame False {
            # "#BugFixSpracheRegisterkarten"
            n194 = property class="Seite"(reference=w527, error in=w524, "IndependentLabel"=TRUE ("Unabhängige Beschriftung"), "TabCaption"=w523) -> (reference out=w526:refnum<vi>, error out=w525:errorcluster)
          }
          frame True {
          }
        }
      }
      n195 = Close Reference(reference=w503, error in (no error)=w502) -> (error out=w500:errorcluster)
    }
    frame 83 {
      w536 = refnum<vi> refnum  # XYGraph
      w540 = 100
      w552 = refnum<vi> refnum  # Allgemein
      # "#BugFix73"
      n196 = To More Generic Class(target class=w552, reference=w530) -> (generic class reference=w551:refnum<vi>)
      n197 = To More Specific Class(target class=w536, reference=w551, error in=w535) -> (specific class reference=w550:refnum<vi>, error out=w549:errorcluster)
      n198 = property class="XYGraph"(reference=w550, error in=w549) -> (reference out=w543:refnum<vi>, error out=w548:errorcluster, "XScale.NameLbl.Text"=w544:string)
      n199 = call "Namen aus Tabelle ersetzen.vi"("Regulärer Ausdruck"=w544, "Sprachauswahl"=w531, "Tabelle"=w534) -> ("Übersetzung"=w541:string)  [unwired: 7 in, 1 out]
      n200 = Empty String/Path?(string/path=w541) -> (empty?=w542:bool)
      n201 = for {
        N: w540 -> [_]
        tunnel: w543 -> [w573]
        tunnel: w548 -> [w570]
        tunnel: w534 -> [w569]
        tunnel: w531 -> [w568]
        tunnel: [w564] -> _
        tunnel: [w563] -> w538
        tunnel: [w561] -> w545 mode=indexing
        i -> [w572]
        stop <- w559 stop-if-true
        n202 = property class="XYGraph"(reference=w573, error in=w570, "Active Plot"=w572) -> (reference out=w571:refnum<vi>, error out=w558:errorcluster)
        n203 = property class="XYGraph"(reference=w571, error in=w558) -> (reference out=w567:refnum<vi>, error out=w566:errorcluster, "Plot.Plot Name"=w561:string)
        n204 = call "Namen aus Tabelle ersetzen.vi"("Regulärer Ausdruck"=w561, "Sprachauswahl"=w568, "Tabelle"=w569) -> ("Übersetzung"=w562:string)  [unwired: 7 in, 1 out]
        n205 = Empty String/Path?(string/path=w562) -> (empty?=w565:bool)
        n206 = case shown="False" w565 {
          tunnel: w567 -> [w578 w580]
          tunnel: w566 -> [w577 w579]
          tunnel: [w576 w580] -> w564
          tunnel: [w575 w579] -> w563
          tunnel: w562 -> [w574 _]
          frame False {
            n207 = property class="XYGraph"(reference=w578, error in=w577, "Plot.Plot Name"=w574) -> (reference out=w576:refnum<vi>, error out=w575:errorcluster)
          }
          frame True {
          }
        }
        n208 = call <vilib>:"Clear Errors.vi"("error in (no error)"=w558, "specific error code to clear (0: all)"=1077) -> ("error out"=w559:errorcluster)  [unwired: 4 in, 1 out]
      }
      n209 = for {
        N: w540 -> [_]
        tunnel: w534 -> [w594]
        tunnel: w531 -> [w589]
        tunnel: w543 -> [w587]
        tunnel: w548 -> [w588]
        tunnel: [w591] -> w547
        tunnel: [w590] -> w546
        i -> [w585]
        stop <- w583 stop-if-true
        n210 = property class="XYGraph"(reference=w587, error in=w588, "ActYScl"=w585) -> (reference out=w586:refnum<vi>, error out=w582:errorcluster, "YScale.NameLbl.Text"=w584:string)
        n211 = call "Namen aus Tabelle ersetzen.vi"("Regulärer Ausdruck"=w584, "Sprachauswahl"=w589, "Tabelle"=w594) -> ("Übersetzung"=w592:string)  [unwired: 7 in, 1 out]
        n212 = Empty String/Path?(string/path=w592) -> (empty?=w593:bool)
        n213 = case shown="False" w593 {
          tunnel: w582 -> [w599 w600]
          tunnel: w586 -> [w598 w601]
          tunnel: [w597 w600] -> w590
          tunnel: [w596 w601] -> w591
          tunnel: w592 -> [w595 _]
          frame False {
            n214 = property class="XYGraph"(reference=w598, error in=w599, "YScale.NameLbl.Text"=w595) -> (reference out=w596:refnum<vi>, error out=w597:errorcluster)
          }
          frame True {
          }
        }
        n215 = call <vilib>:"Clear Errors.vi"("error in (no error)"=w582, "specific error code to clear (0: all)"=1077) -> ("error out"=w583:errorcluster)  [unwired: 4 in, 1 out]
      }
      n216 = case shown="False" w542 {
        tunnel: w543 -> [w556 w557]
        tunnel: [w555 _] -> w537
        tunnel: [w554 w557] -> _
        tunnel: w541 -> [w553 _]
        frame False {
          n217 = property class="XYGraph"(reference=w556, "XScale.NameLbl.Text"=w553) -> (reference out=w554:refnum<vi>, error out=w555:errorcluster)  [unwired: 1 in]
        }
        frame True {
        }
      }
      n218 = Merge Errors(w537, w546, w538) -> (w539:errorcluster)
      n219 = Build Array (concatenate)(w544, w545) -> (w533:string[])
      n220 = Close Reference(reference=w547, error in (no error)=w539) -> (error out=w532:errorcluster)
    }
  }
  "Strings [4]" <- w9
  "Cluster Elemente[]" <- w3
  n221 = call <vilib>:"Clear Errors.vi"("error in (no error)"=w2) -> ("error out"=→"error out":errorcluster)  [unwired: 5 in, 1 out]
  "Sprachauswahl out" <- "Sprachauswahl"
  "ClassID out" <- "ClassID"
  "all rows out" <- "all rows"
